vi "startUp.vi"(8 "error in (no error)":errorcluster, 10 "ScriptEvent":refnum<class "ScriptEvent.lvclass">, 11 "SingleToneRampAction in":refnum<class "SingleToneRampAction.lvclass">) -> (0 "error out":errorcluster, 3 "SingleToneRampAction out":refnum<class "SingleToneRampAction.lvclass">)   [LabVIEW 2011, in "Views.lvlib" / "ScriptEditor.lvlib" / "SingleToneRampAction.lvclass"]
uses:
  SingleToneRampAction.lvclass
  Tools/Scripting/ScriptingEvent/ScriptEvent.lvclass
  Tools/Scripting/ScriptingEvent/ScriptEvents/SingleTone/SingleToneRamp/SingleToneRamp.lvclass
  SingleToneRampAction.lvclass/SingleToneRampAction.ctl
  ActionPanel.lvclass
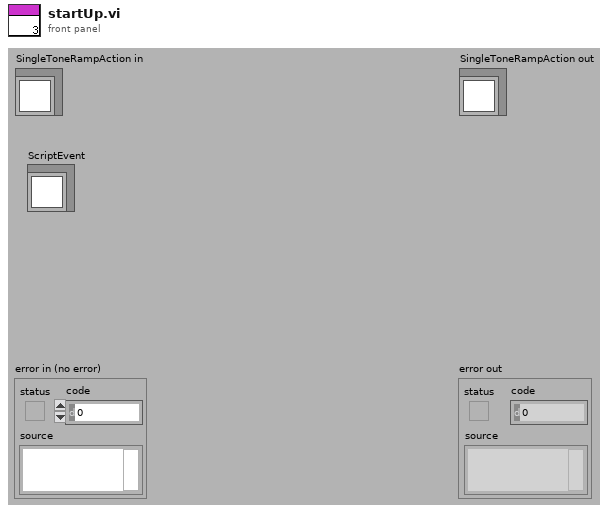
[diagram p1: front panel]
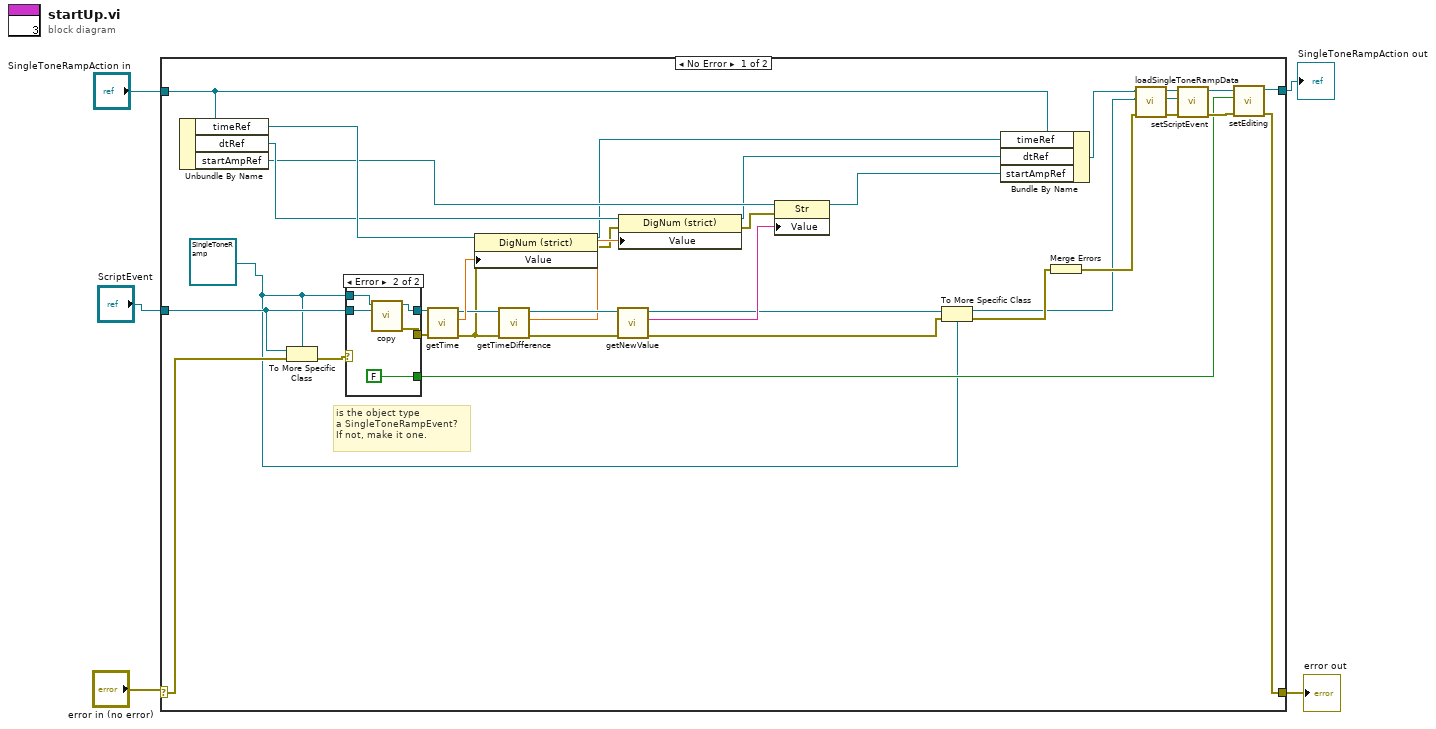
[diagram p0: block diagram]
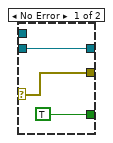
[diagram p2: hidden frame]
diagram:
  n1 = case shown="No Error" "error in (no error)" {
    selector: "error in (no error)" -> [w22 w51]
    tunnel: [w18 w51] -> w2
    tunnel: [w20 w50] -> w1
    tunnel: "SingleToneRampAction in" -> [w16 w50]
    tunnel: "ScriptEvent" -> [w38 _]
    frame No Error {
      w8 = refnum<class "SingleToneRamp.lvclass"> refnum ("Tools.lvlib:Scripting.lvlib:SingleToneRamp.lvclass")
      # "is the object type\na SingleToneRampEvent?\nIf not, make it one."
      n2 = Unbundle By Name(w16) -> ("timeRef"=w37:refnum<vi>, "dtRef"=w36:refnum<vi>, "startAmpRef"=w35:refnum<vi>)
      n3 = To More Specific Class(target class=w8, reference=w38, error in=w22) -> (error out=w41:errorcluster)  [unwired: 1 out]
      n4 = case shown="Error" w41 {
        selector: w41 -> [w43 _]
        tunnel: w38 -> [w44 w48]
        tunnel: w8 -> [_ w49]
        tunnel: [w43 w47] -> w40
        tunnel: [w44 w46] -> w39
        tunnel: [TRUE FALSE] -> w17
        frame No Error {
        }
        frame Error {
          n5 = call-dynamic "copy.vi"("ScriptEventForCopy"=w48, "SingleToneRamp in"=w49) -> ("error out"=w47:errorcluster, "SingleToneRamp Copy"=w46:refnum<class "SingleToneRamp.lvclass">)  [unwired: 8 in]
        }
      }
      n6 = call "getTime.vi"("error in (no error)"=w40, "ScriptEvent.lvclass in"=w39) -> ("error out"=w28:errorcluster, "time"=w34:dbl, "ScriptEvent.lvclass out"=w33:refnum<class "ScriptEvent.lvclass">)  [unwired: 7 in]
      n7 = property class="DigNum (strict)"(reference=w37, error in=w28, "Value"=w34) -> (reference out=w25:refnum<vi>, error out=w27:errorcluster)
      n8 = call "getTimeDifference.vi"("error in (no error)"=w28, "ScriptEvent.lvclass in"=w33) -> ("error out"=w29:errorcluster, "time difference"=w31:dbl, "ScriptEvent.lvclass out"=w32:refnum<class "ScriptEvent.lvclass">)  [unwired: 7 in]
      n9 = call "getNewValue.vi"("error in (no error)"=w29, "ScriptEvent.lvclass in"=w32) -> ("error out"=w14:errorcluster, "newValue"=w30:string, "ScriptEvent.lvclass out"=w15:refnum<class "ScriptEvent.lvclass">)  [unwired: 7 in]
      n10 = property class="DigNum (strict)"(reference=w36, error in=w27, "Value"=w31) -> (reference out=w24:refnum<vi>, error out=w26:errorcluster)
      n11 = property class="Str"(reference=w35, error in=w26, "Value"=w30) -> (reference out=w13:refnum<vi>)  [unwired: 1 out]
      n12 = To More Specific Class(target class=w8, reference=w15, error in=w14) -> (specific class reference=w7:refnum<class "SingleToneRamp.lvclass">, error out=w23:errorcluster)
      n13 = Bundle By Name(cluster=w16, "timeRef"=w25, "dtRef"=w24, "startAmpRef"=w13) -> (w11:refnum<class "SingleToneRampAction.lvclass">)
      n14 = Merge Errors(w23) -> (w10:errorcluster)
      n15 = call "loadSingleToneRampData.vi"("error in (no error)"=w10, "toneRamp"=w7, "SingleToneRampAction in"=w11) -> ("error out"=w9:errorcluster, "toneRampOut"=w6:refnum<class "SingleToneRamp.lvclass">, "SingleToneRampAction out"=w12:refnum<class "SingleToneRampAction.lvclass">)  [unwired: 6 in]
      n16 = call "setScriptEvent.vi"("error in (no error)"=w9, "ScriptEvent.lvclass"=w6, "ActionPanel.lvclass in"=w12) -> ("error out"=w19:errorcluster, "ActionPanel.lvclass out"=w21:refnum<class "SingleToneRampAction.lvclass">)  [unwired: 7 in]
      n17 = call "setEditing.vi"("error in (no error)"=w19, "editing?"=w17, "ActionPanel.lvclass in"=w21) -> ("error out"=w18:errorcluster, "ActionPanel.lvclass out"=w20:refnum<class "SingleToneRampAction.lvclass">)  [unwired: 7 in]
    }
    frame Error {
    }
  }
  "error out" <- w2
  "SingleToneRampAction out" <- w1
